vi "Interface_Asset_Initalize Assets.vi"(8 "error in (no error)":errorcluster, 11 "Grid in":refnum<class "Grid.lvclass">) -> (0 "error out":errorcluster, 2 "TagDescriptions":refnum<class "tag descriptor.lvclass">[](array[class]), 3 "Grid out":refnum<class "Grid.lvclass">)   [LabVIEW 2015, in "Grid.lvclass"]
uses:
  Grid.lvclass
  <vilib>/NI/Tag Bus/tag/tag descriptor.lvclass
  TagBus/TagBus.lvclass
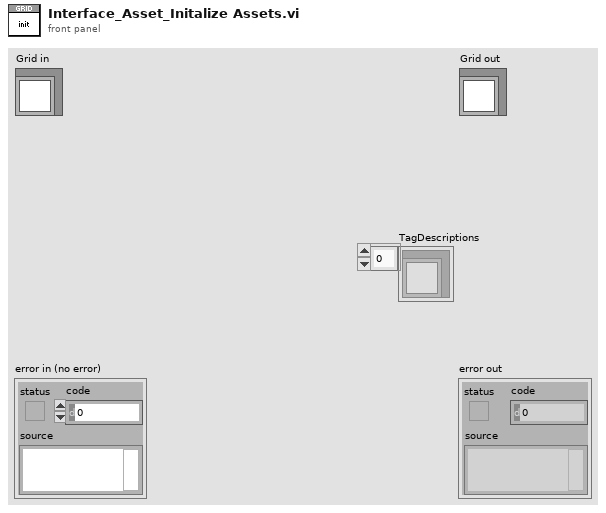
[diagram p1: front panel]
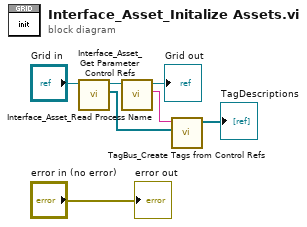
[diagram p0: block diagram]
diagram:
  n1 = call-dynamic "Interface_Asset_Get Parameter Control Refs.vi"("Grid in"="Grid in") -> ("Controls[]"=w1:refnum<vi>[], "Grid out"=w2:refnum<class "Grid.lvclass">)  [unwired: 8 in, 1 out]
  n2 = call-dynamic "Interface_Asset_Read Process Name.vi"("Grid in"=w2) -> ("Process Name"=w5:string, "Grid out"=→"Grid out":refnum<class "Grid.lvclass">)  [unwired: 9 in]
  n3 = call "TagBus_Create Tags from Control Refs.vi"("Array"=w1, "Prepend Tag Name"=w5) -> ("TagDescriptions"=→"TagDescriptions":refnum<class "tag descriptor.lvclass">[])  [unwired: 9 in]
  "error out" <- "error in (no error)"
